vi "SenderLoop.vi"(10 "IP Address":string="localhost", 11 "name":string="command") -> ()   [LabVIEW 2014]
uses:
  CommMsg.ctl
  CommState.ctl
panel:
  out "end":bool
  in  "variant":variant
  out "error out":errorcluster
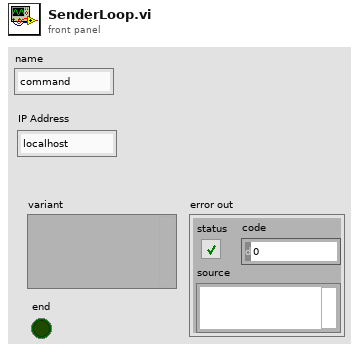
[diagram p1: front panel]
types:
  T1 = typedef "CommState.ctl" = enum16{"Disconnected", "Connected"}
  T2 = typedef "CommMsg.ctl" = cluster{"cmd":enum16{"exit", "data"}, "value":variant}
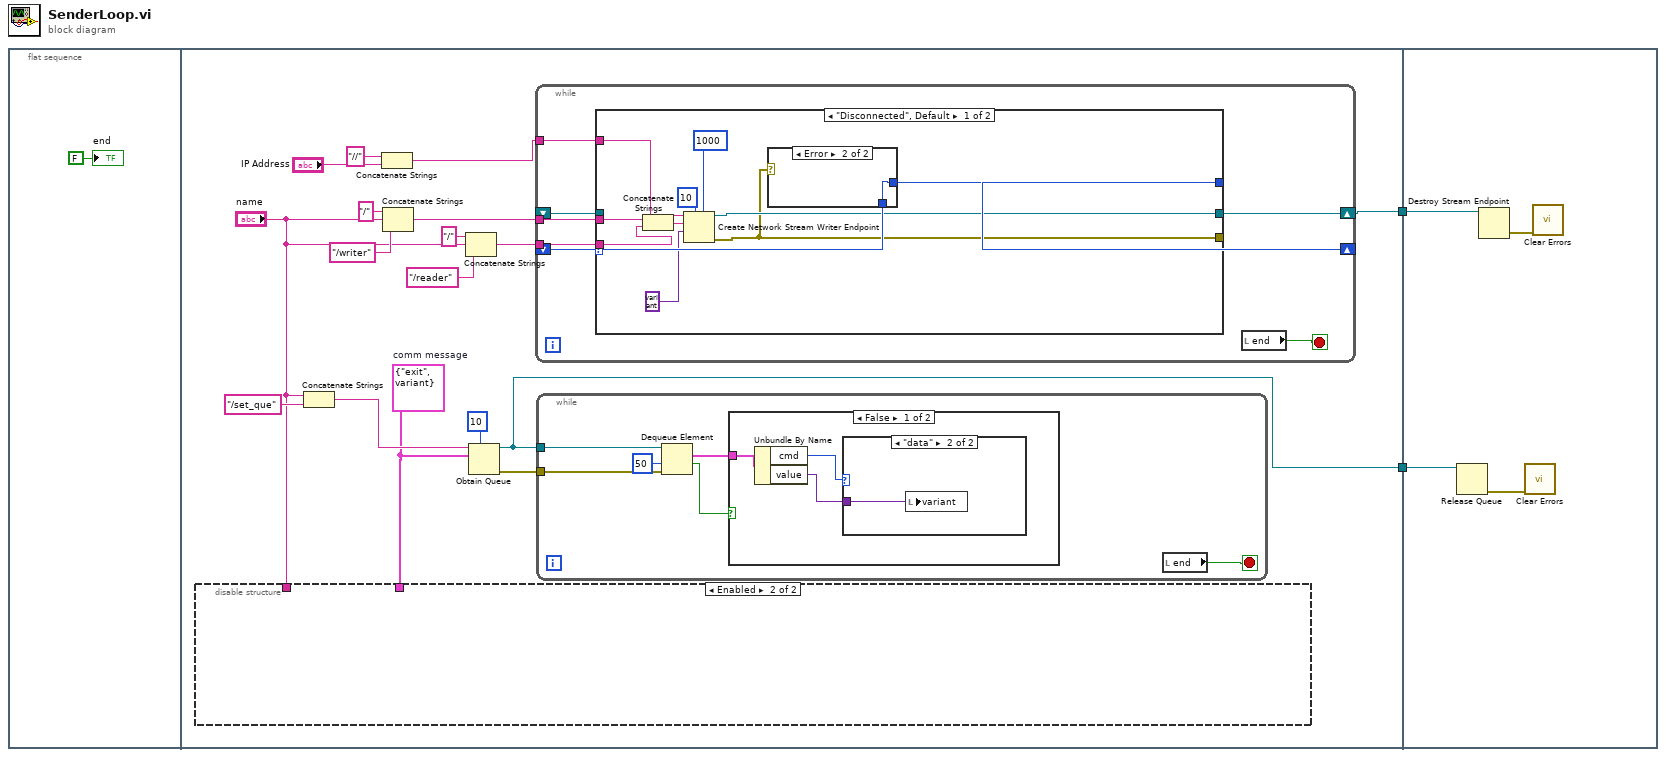
[diagram p0: block diagram]
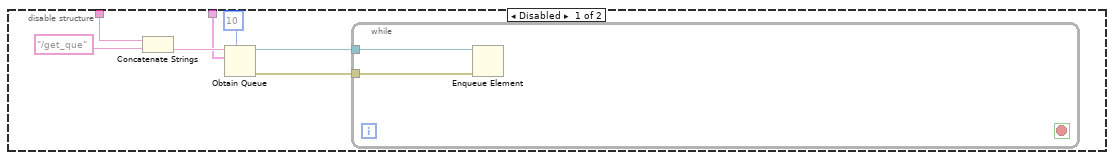
[diagram p2: hidden frame]
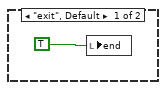
[diagram p3: hidden frame]
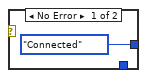
[diagram p5: hidden frame]
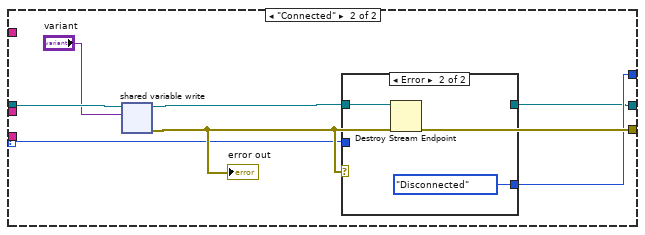
[diagram p6: hidden frame]
diagram:
  n1 = flat-sequence {
    tunnel: [w6] -> w2
    tunnel: [w5] -> w1
    tunnel: w2 -> [w76]
    tunnel: w1 -> [w75]
    frame #0 {
      "end" <- FALSE ("end")
    }
    frame #1 {
      w7 = T2 {"cmd"=enum."exit", "value"=variant}  # comm message
      n2 = disable-structure shown="Enabled" {
        disable-tunnel: "name" -> [w26 _]
        disable-tunnel: w7 -> [w23 _]
        frame Disabled {
          n3 = Concatenate Strings(w26, "/get_que" ("writer name")) -> (w27:string)
          n4 = Obtain Queue(max queue size (-1, unlimited)=10, name (unnamed)=w27, element data type=w23) -> (queue out=w24:refnum<queue>, error out=w21:errorcluster)  [unwired: 2 in, 1 out]
          n5 = while {
            tunnel: w24 -> [w29]
            tunnel: w21 -> [w28]
            stop <- _ stop-if-true
            n6 = Enqueue Element(queue=w29, error in (no error)=w28) -> ()  [unwired: 2 in, 3 out]
          }
        }
        frame Enabled {
        }
      }
      n7 = Concatenate Strings("name", "/set_que" ("writer name")) -> (w8:string)
      n8 = Concatenate Strings("//" ("reader url"), "IP Address") -> (w18:string)
      n9 = Concatenate Strings("/" ("string"), "name", "/writer" ("writer name")) -> (w13:string)
      n10 = Concatenate Strings("/" ("string"), "name", "/reader" ("writer name")) -> (w12:string)
      n11 = Obtain Queue(max queue size (-1, unlimited)=10, name (unnamed)=w8, element data type=w7) -> (queue out=w6:refnum<queue>, error out=w10:errorcluster)  [unwired: 2 in, 1 out]
      n12 = while {
        tunnel: w18 -> [w47]
        shift-right: [w46] -> w5
        shift-left: _ -> [w45]
        shift-right: [w44] -> _
        shift-left: _ -> [w48]
        tunnel: w13 -> [w43]
        tunnel: w12 -> [w42]
        stop <- w41 stop-if-true
        n13 = case shown="\"Disconnected\", Default" w48 {
          selector: w48 -> [w57 w65]
          tunnel: w47 -> [w59 _]
          tunnel: [w56 w63] -> w46
          tunnel: w45 -> [_ w68]
          tunnel: [w55 w67] -> _
          tunnel: [w58 w66] -> w44
          tunnel: w43 -> [w51 _]
          tunnel: w42 -> [w50 _]
          frame "Disconnected", Default {
            n14 = Concatenate Strings(w59, w50) -> (w54:string)
            n15 = Create Network Stream Writer Endpoint(5:1000 ("timeout in ms (-1)"), 7:10 ("reader buffer size"), 9:variant ("variant"), 10:w54, 11:w51) -> (0:w55:errorcluster, 3:w56:refnum<k21>)  [unwired: 2 in]
            n16 = case shown="Error" w55 {
              tunnel: [CommState."Connected" ("comm state") w61] -> w58
              tunnel: w57 -> [_ w61]
              frame No Error {
              }
              frame Error {
              }
            }
          }
          frame "Connected" {
            n17 = shared-variable-write(w68, "variant") -> (w64:refnum<k21>, w67:errorcluster)  [unwired: 2 in, 1 out]
            "error out" <- w67
            n18 = case shown="Error" w67 {
              tunnel: w65 -> [w70 _]
              tunnel: [w70 CommState."Disconnected" ("comm state")] -> w66
              tunnel: w64 -> [w69 w71]
              tunnel: [w69 _] -> w63
              frame No Error {
              }
              frame Error {
                n19 = Destroy Stream Endpoint(11:w71) -> ()  [unwired: 1 in, 1 out]
              }
            }
          }
        }
        n20 = local read "end"() -> (w41:bool)
      }
      n21 = while {
        tunnel: w6 -> [w35]
        tunnel: w10 -> [w34]
        stop <- w30 stop-if-true
        n22 = Dequeue Element(queue=w35, timeout in ms (-1)=50, error in (no error)=w34) -> (element=w31:T2, timed out?=w32:bool)  [unwired: 2 out]
        n23 = case shown="False" w32 {
          tunnel: w31 -> [w38 _]
          frame False {
            n24 = Unbundle By Name(w38) -> ("cmd"=w37:enum16{"exit", "data"}, "value"=w36:variant)
            n25 = case shown="\"data\"" w37 {
              tunnel: w36 -> [_ w40]
              frame "exit", Default {
                n26 = local write "end"(TRUE ("stop")) -> ()
              }
              frame "data" {
                n27 = local write "variant"(w40) -> ()
              }
            }
          }
          frame True {
          }
        }
        n28 = local read "end"() -> (w30:bool)
      }
    }
    frame #2 {
      n29 = Release Queue(queue=w76) -> (error out=w73:errorcluster)  [unwired: 2 in, 2 out]
      n30 = Destroy Stream Endpoint(11:w75) -> (0:w74:errorcluster)  [unwired: 1 in]
      n31 = call <vilib>:"Clear Errors.vi"("error in (no error)"=w73) -> ()  [unwired: 5 in, 2 out]
      n32 = call <vilib>:"Clear Errors.vi"("error in (no error)"=w74) -> ()  [unwired: 5 in, 2 out]
    }
  }
